vi "Close.vi"(8 "error in (no error)":errorcluster, 11 "VectoService in":refnum<class "VectoInfo.lvclass">) -> (0 "error out":errorcluster)   [LabVIEW 2020, in "Vecto.lvlib" / "VectoInfo.lvclass"]
uses:
  VectoInfo.lvclass
  VectoInfo.lvclass/VectoInfo.ctl
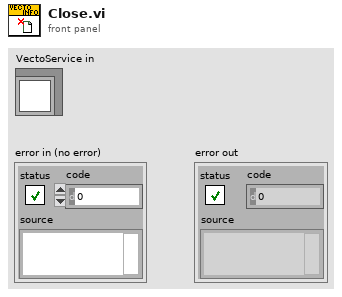
[diagram p1: front panel]
types:
  T1 = typedef "Vecto.lvlib/VectoInfo.lvclass/Incoming Events.ctl" = cluster{"Request Info":refnum<user-event>, "Update Connection":refnum<user-event>, "Update Info":refnum<user-event>, "Close":refnum<user-event>, "Remove Connection":refnum<user-event>, "Add RX":refnum<user-event>, "Add TX":refnum<user-event>}
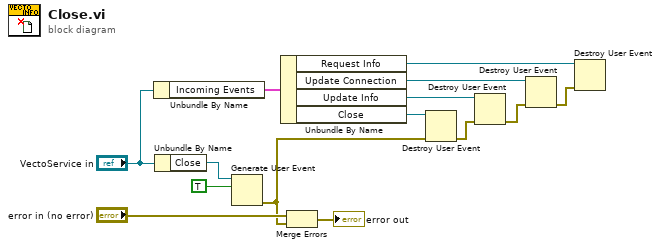
[diagram p0: block diagram]
diagram:
  n1 = Unbundle By Name("VectoService in") -> ("Incoming Events"=w9:T1)
  n2 = Unbundle By Name("VectoService in") -> ("Close"=w14:refnum<user-event>)
  n3 = Generate User Event(user event=w14, event data cluster=TRUE ("event data")) -> (error out=w7:errorcluster)  [unwired: 2 in, 1 out]
  n4 = Unbundle By Name(w9) -> ("Request Info"=w1:refnum<user-event>, "Update Connection"=w3:refnum<user-event>, "Update Info"=w6:refnum<user-event>, "Close"=w8:refnum<user-event>)
  n5 = Merge Errors("error in (no error)", w7) -> (→"error out":errorcluster)
  n6 = Destroy User Event(user event=w8, error in=w7) -> (error out=w5:errorcluster)
  n7 = Destroy User Event(user event=w6, error in=w5) -> (error out=w2:errorcluster)
  n8 = Destroy User Event(user event=w3, error in=w2) -> (error out=w4:errorcluster)
  n9 = Destroy User Event(user event=w1, error in=w4) -> ()  [unwired: 1 out]
